vi "Inst.RP100.setLevel.vi"(8 "error in (no error)":errorcluster, 10 "Variant":variant, 11 "Inst.RP100 out":refnum<class "Inst.RP100.lvclass">) -> (0 "error out":errorcluster, 3 "Inst.RP100 out":refnum<class "Inst.RP100.lvclass">)   [LabVIEW 2019, in "Inst.RP100.lvclass"]
uses:
  Inst.RP100.lvclass
  Typedefs/Output State--Enum.ctl
  Typedefs/setLevel--Cluster.ctl
  Typedefs/Output Channel--Enum.ctl
  Inst.RP100.lvclass/Inst.RP100.ctl
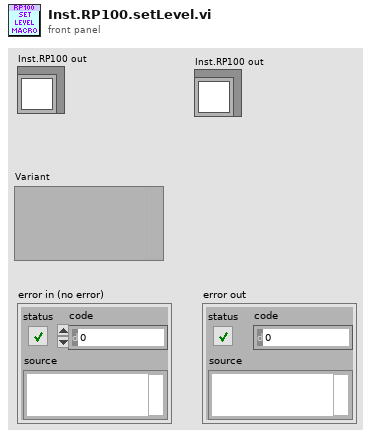
[diagram p1: front panel]
types:
  T1 = typedef "Inst.RP100.lvclass/setLevel--Cluster.ctl" = cluster{"Output Channel":T2, "Level (V)":dbl, "Slew (V/s)":dbl}
  T2 = typedef "Inst.RP100.lvclass/Output Channel--Enum.ctl" = enum16{"Output 1", "Output 2"}
  T3 = typedef "Inst.RP100.lvclass/Output State--Enum.ctl" = enum16{"Shorted", "Enabled"}
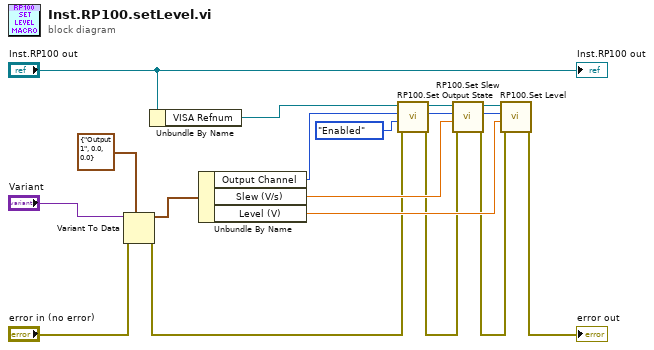
[diagram p0: block diagram]
diagram:
  n1 = Variant To Data(error in="error in (no error)", type=T1 {"Output Channel"=enum."Output 1", "Level (V)"=0.0, "Slew (V/s)"=0.0} ("Data in"), Variant="Variant") -> (data=w7:T1, error out=w4:errorcluster)
  n2 = Unbundle By Name("Inst.RP100 out") -> ("VISA Refnum"=w3:refnum<visa-resource-name>)
  n3 = Unbundle By Name(w7) -> ("Output Channel"=w17:T2, "Slew (V/s)"=w16:dbl, "Level (V)"=w18:dbl)
  n4 = call "RP100.Set Output State.vi"("error in (no error)"=w4, "Output State"=Output_State--Enum."Enabled", "Output Channel"=w17, "VISA resource name"=w3) -> ("error out"=w9:errorcluster, "Output Channel"=w13:T2, "VISA Refnum out"=w12:refnum<visa-resource-name>)  [unwired: 5 in]
  n5 = call "RP100.Set Slew.vi"("error in (no error)"=w9, "Slew (V/s)"=w16, "Output Channel"=w13, "VISA resource name"=w12) -> ("error out"=w10:errorcluster, "Output Channel"=w14:T2, "VISA Refnum out"=w15:refnum<visa-resource-name>)  [unwired: 5 in]
  n6 = call "RP100.Set Level.vi"("error in (no error)"=w10, "Level (V)"=w18, "Output Channel"=w14, "VISA resource name"=w15) -> ("error out"=→"error out":errorcluster)  [unwired: 5 in, 2 out]
  "Inst.RP100 out" <- "Inst.RP100 out"
